vi "DSF.Engine.Interface.RT FIFO.Read.vi"   [LabVIEW 2017, in "DSF.Engine.lvlib" / "DSF.Engine.Interface.lvclass"]
uses:
  DSF.Engine.Interface.lvclass
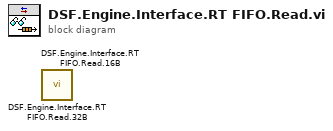
[diagram p0: block diagram]
diagram:
  n1 = call "DSF.Engine.Interface.RT FIFO.Read.32B.vi"() -> ()  [unwired: 7 in, 5 out]
  n2 = call "DSF.Engine.Interface.RT FIFO.Read.16B.vi"() -> ()  [unwired: 7 in, 5 out]
